vi "ELVIS III v1.0 Block Write DMA.vi"   [LabVIEW 2021]
uses:
  <vilib>/Platform/TimedLoop/XDataNode/timing_clust.ctl
  <vilib>/Platform/TimedLoop/XDataNode/nitl_modes.ctl
  <vilib>/Platform/TimedLoop/XDataNode/wakeup.ctl
  <vilib>/myRIO/Common/Instrument Driver Framework/Utilities/typedefs/FPGA Ref Manager Action Enum.ctl
  <vilib>/myRIO/Common/Instrument Driver Framework/ELVIS III v1.0/DO Block/typedefs/ELVIS III DO Block FPGA Reference.ctl
  <vilib>/myRIO/Common/Instrument Driver Framework/ELVIS III v1.0/AO Block/typedefs/ELVIS III AO Block Channels FPGA Reference.ctl
  <vilib>/Utility/error.llb/Error Cluster From Error Code.vi
  <vilib>/rvi/errors/niLvFpgaAdjustHostInterfaceError.vi
  <vilib>/RVI Host/nirviSupport.llb/nirviErrorClusterFromErrorCode.vi
  <vilib>/platform/TimedLoop/XDataNode/XDataNode.xnode
  <vilib>/myRIO/Common/Instrument Driver Framework/Utilities/typedefs/Generic FPGA Reference.ctl
  <vilib>/rvi/interface/nirviReadWriteControl/nirviReadWriteControl.xnode
  <vilib>/rvi/interface/nirviMethod/nirviMethod.xnode
  <vilib>/Platform/TimedLoop/XDataNode/XDNodeRunTimeDep.lvlib
  <vilib>/rvi/interface/nirviMethod/StockFPGA_InlinedMethodWaitForMultipleIRQ.vi
  <vilib>/FPGAPlugInAG/Dynamic/niLvFpga_WaitOnIrq_Dynamic.vi
  NiFpgaLv.dll
  <vilib>/rvi/interface/Simulation/niFpgaSimulationCallBeginRW.vi
  <vilib>/FPGAPlugInAG/Dynamic/niLvFpga_AcknowledgeIrq_Dynamic.vi
types:
  T1 = typedef "Semaphore RefNum" = refnum<k1>
  T2 = typedef "FPGA Ref Manager Action Enum.ctl" = enum16{"Get", "Set", "Reset"}
  T3 = typedef "Generic FPGA Reference.ctl" = refnum<k20>
  T4 = typedef "XDNodeRunTimeDep.lvlib/timing_clust.ctl" = cluster{"Expected End [f-1]":u64, "Actual End [f-1]":u64, "Finished Late? [f-1]":bool, "Expected End [i-1]":u64, "Actual End [i-1]":u64, "Finished Late? [i-1]":bool, "Expected Start [i]":u64, "Actual Start [i]":u64, "Expected Start [f]":u64, "Actual Start [f]":u64, "Source Name":string, "Structure Name":string, "Period":i64, "Deadline":i64, "Offset":i64, "Start":i64, "Priority":i32, "Timeout":i32, "Mode":T5, "Wakeup Reason":T6, "Error":errorcluster, "Source Type":string, "Secondary Source Type":string, "Global End Time":u64, "Global Start Time":u64, "Frame Duration":u64, "Iteration Duration":u64, "Assigned CPU":i32, "I/O Scan Engine Mode":u32}
  T5 = typedef "XDNodeRunTimeDep.lvlib/nitl_modes.ctl" = enum32{"No Change", "Process missed periods, maintain original phase", "Discard missed periods, maintain original phase", "Process missed periods, ignore original phase", "Discard missed periods, ignore original phase"}
  T6 = typedef "XDNodeRunTimeDep.lvlib/wakeup.ctl" = enum32{"Normal", "Aborted", "Asynchronous wakeup", "Timing source error", "Timed loop error", "Timeout"}
  T7 = typedef "ELVIS III DO Block FPGA Reference.ctl" = refnum<k20>
  T8 = typedef "ELVIS III DO Block Configuration.ctl" = cluster{"Wait Until Done?":bool, "DO FIFO Clock Divisor":u16, "Write Mode":u8, "DO (N Samples) Bank Data ":T9[]}
  T9 = typedef "ELVIS III DO Block Bank Data.ctl" = cluster{"Digital Data Reference":refnum<data-value>, "Channel  Bitmask":fxp<+,20,20>, "Semaphore":T1}
  T10 = typedef "ELVIS III AO Block Channels FPGA Reference.ctl" = refnum<k20>
  T11 = typedef "ELVIS III AO Block Configuration.ctl" = cluster{"AO FIFO Clock Divisor":u32, "Wait Until Done?":bool, "Write Mode":u8, "AO (N Samples) Configuration ":T12[]}
  T12 = typedef "ELVIS III AO Block Bank Data.ctl" = cluster{"Analog data reference":refnum<data-value>, "Semaphore":T1, "ENA_MASK":u8}
  T13 = typedef "Block Write Resource.ctl" = refnum<vi>
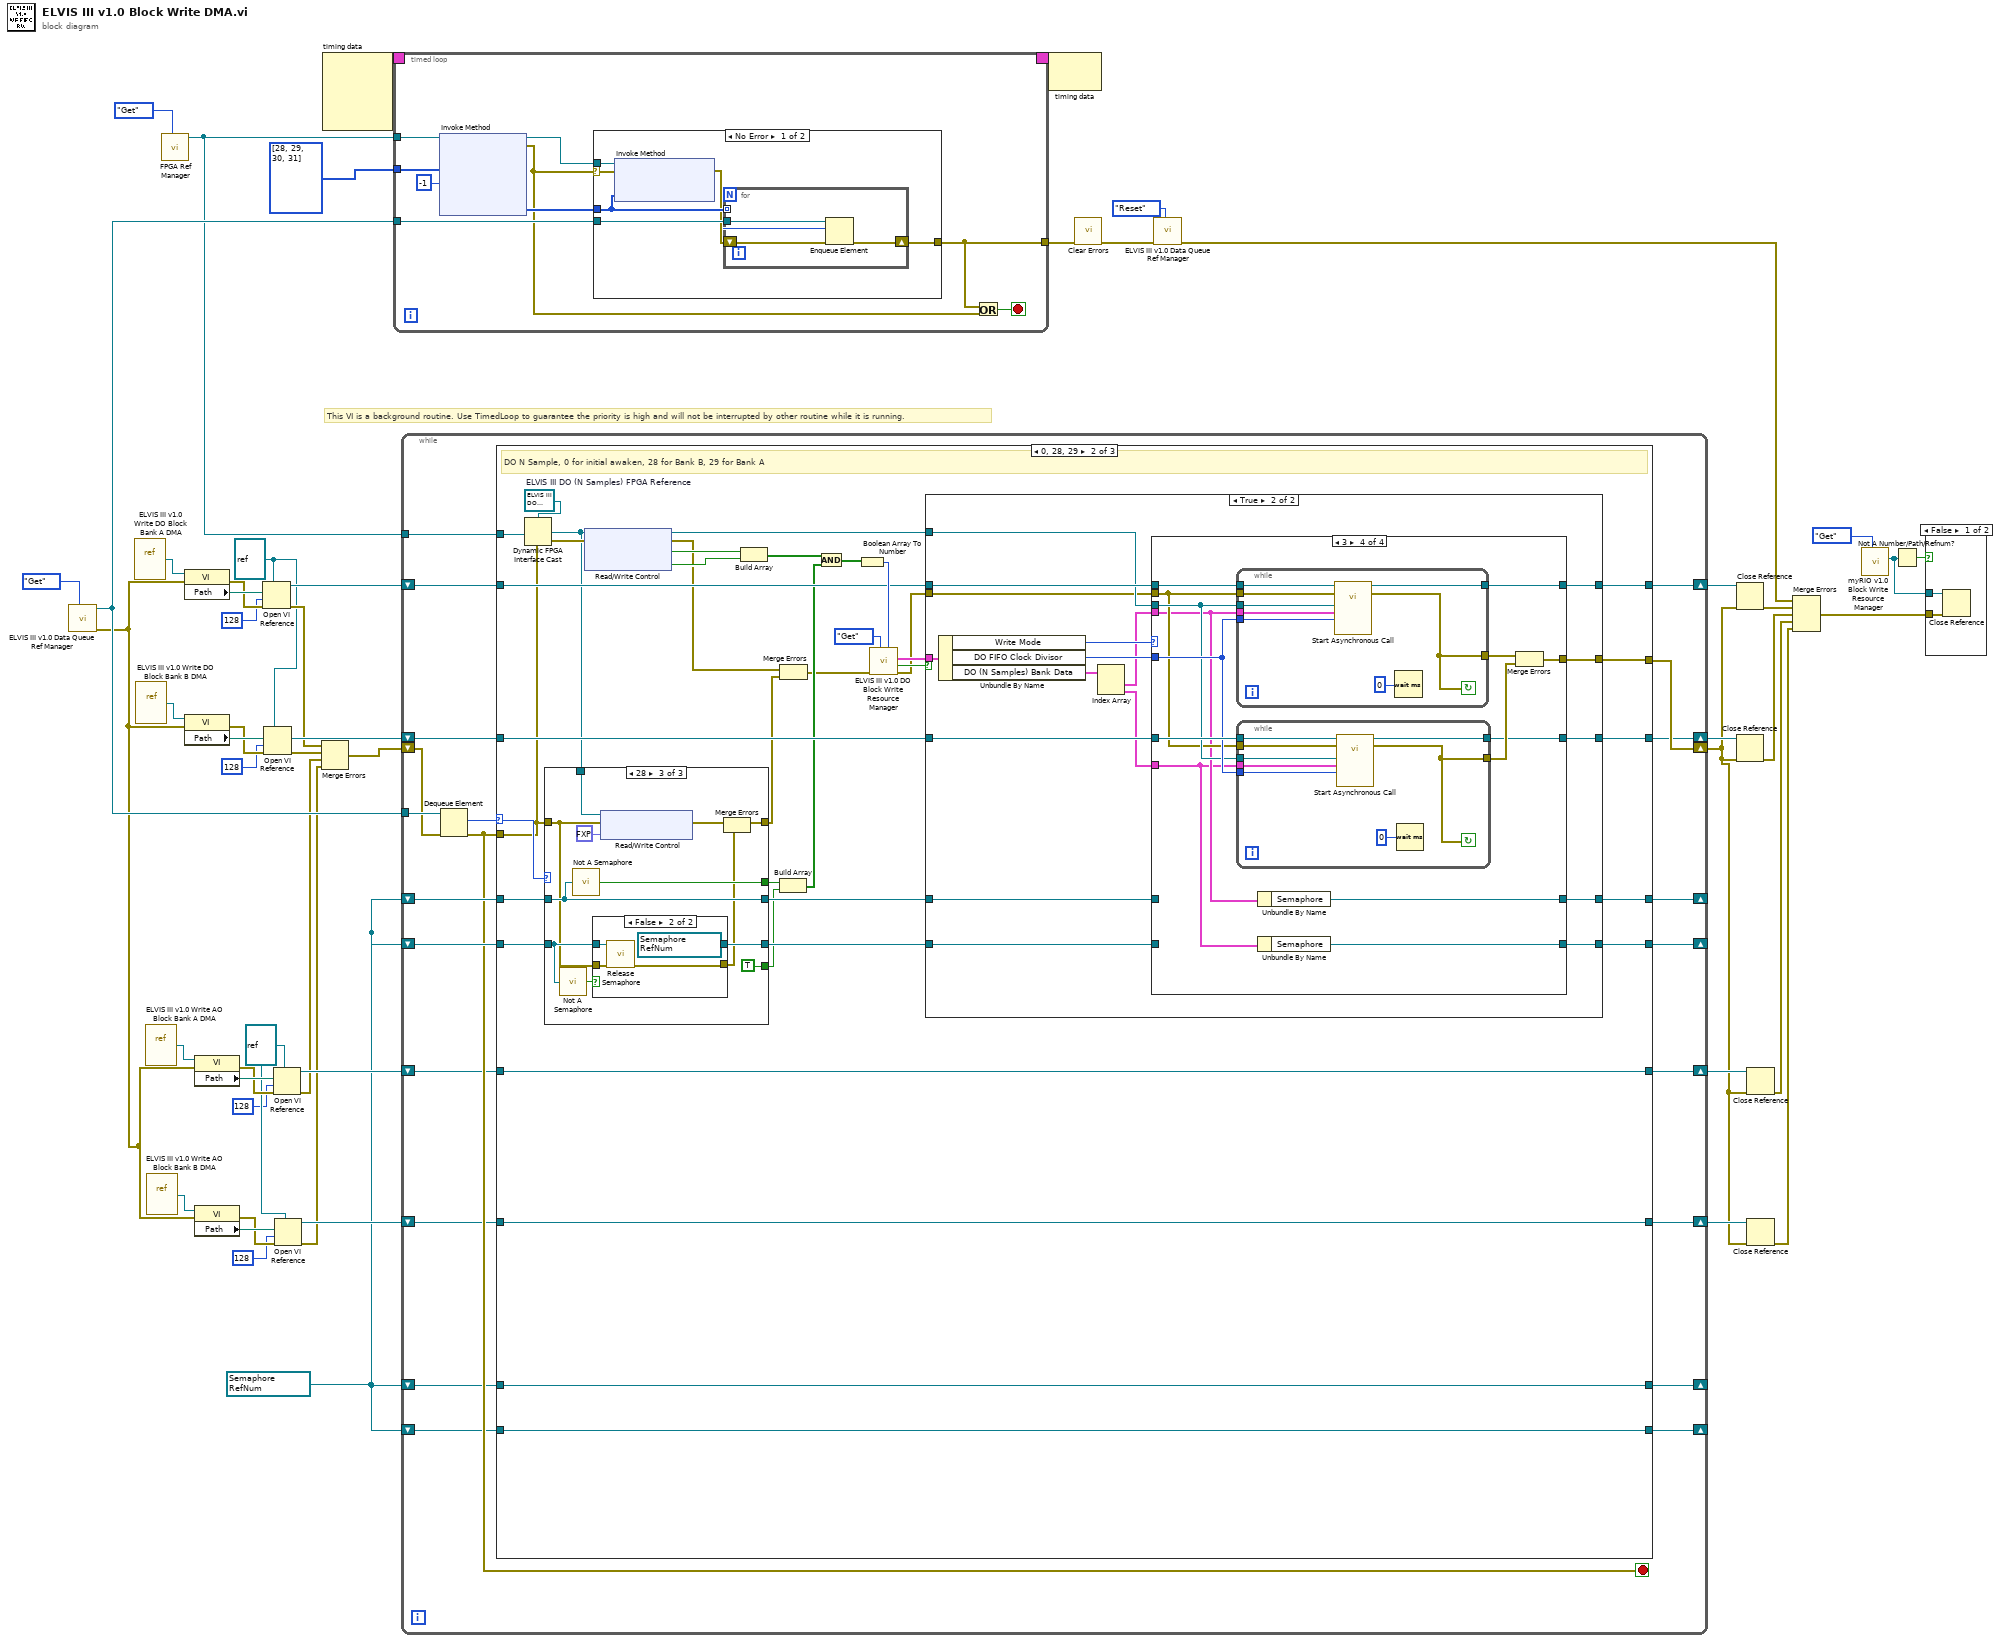
[diagram p0: block diagram]
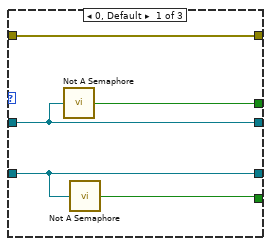
[diagram p4: hidden frame]
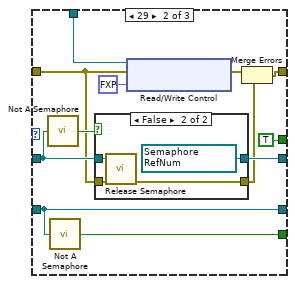
[diagram p5: hidden frame]
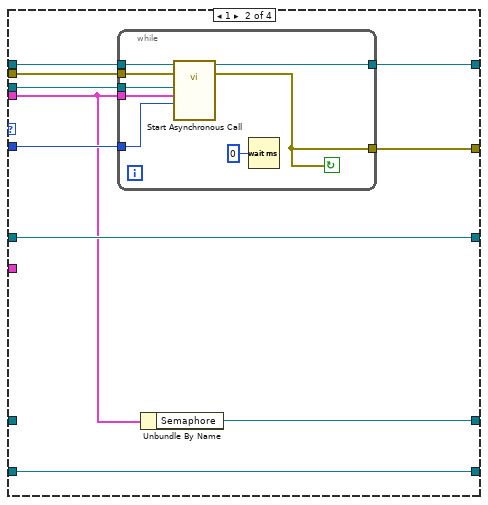
[diagram p10: hidden frame]
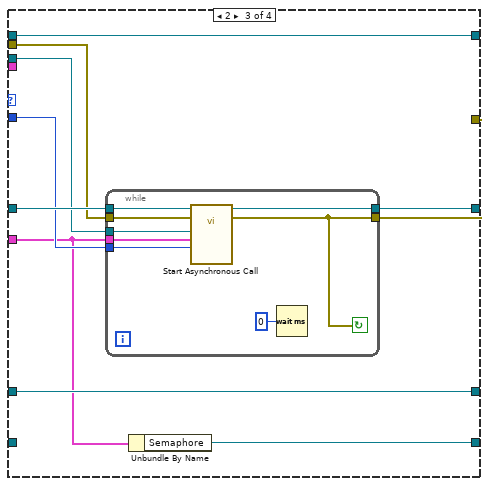
[diagram p11: hidden frame]
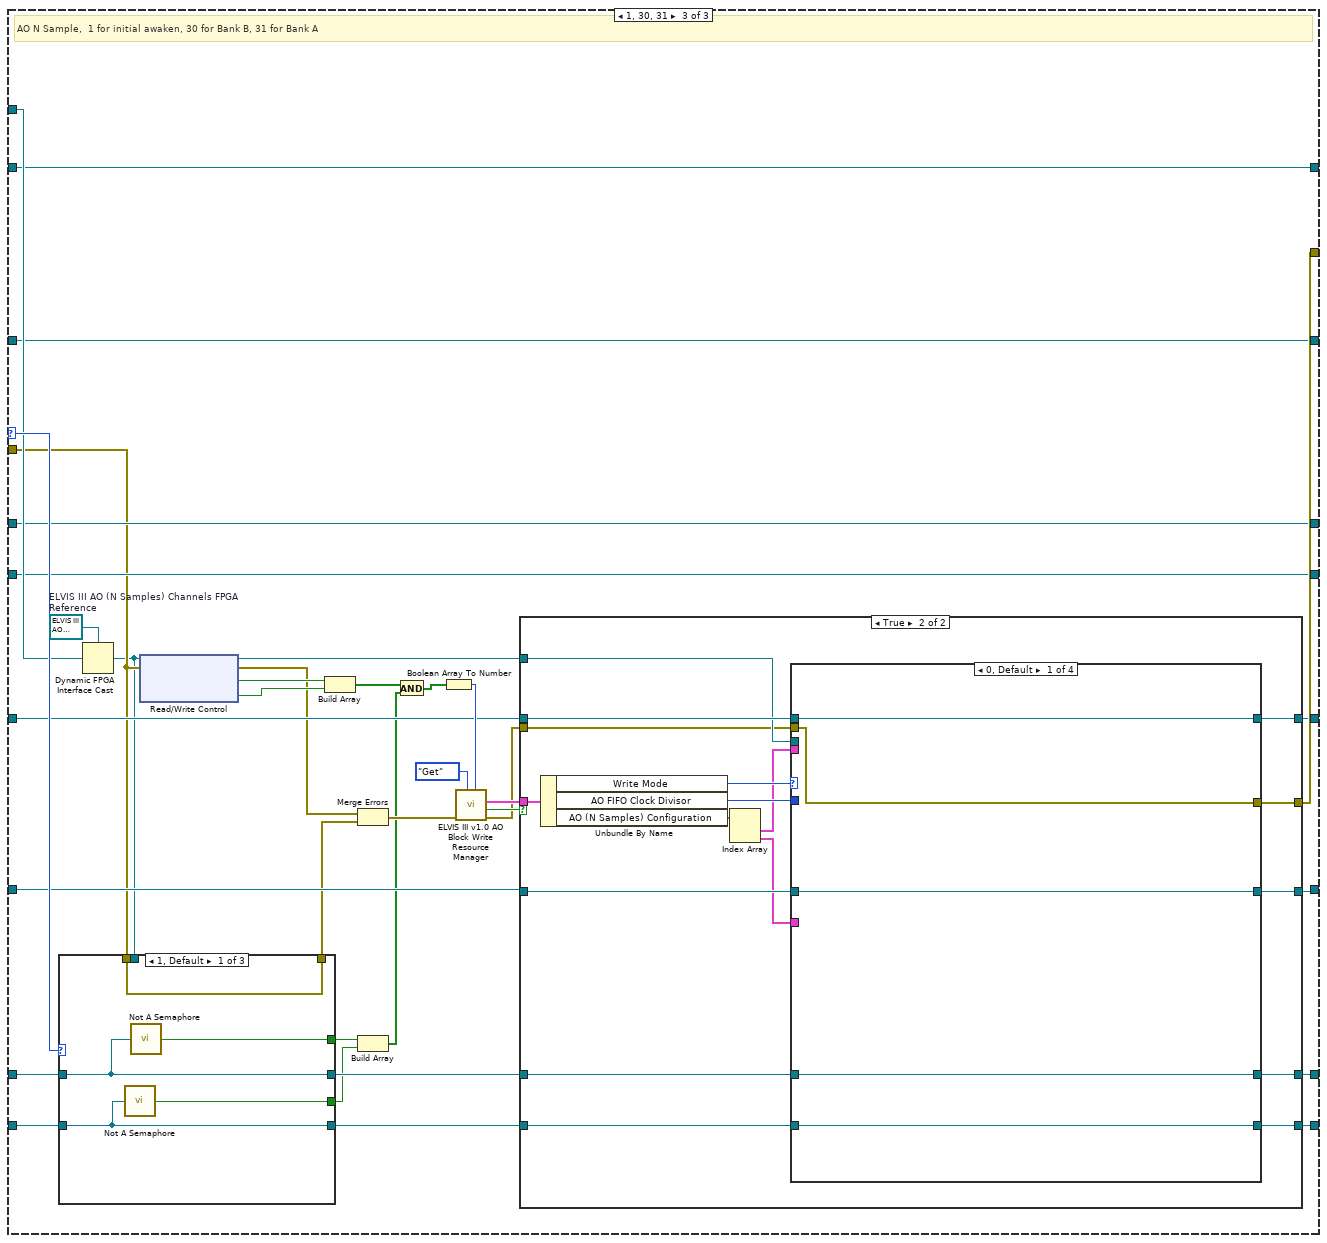
[diagram p12: hidden frame]
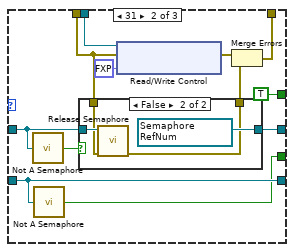
[diagram p13: hidden frame]
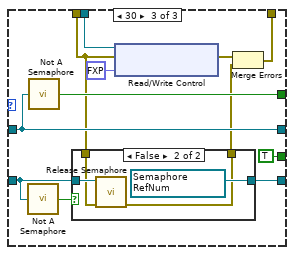
[diagram p15: hidden frame]
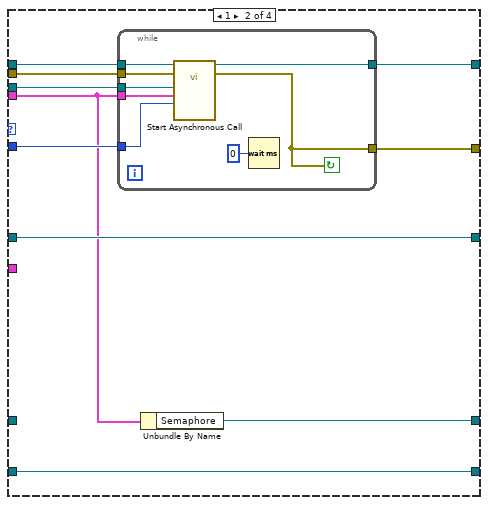
[diagram p18: hidden frame]
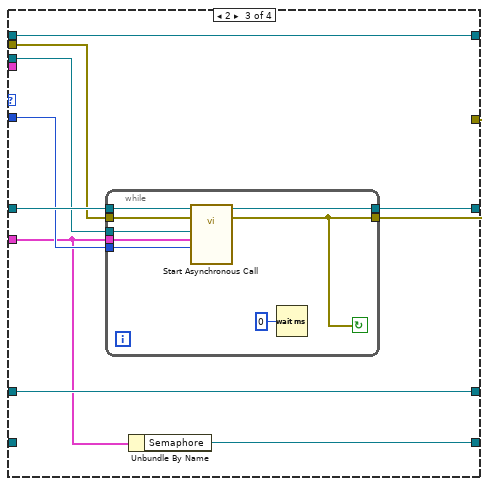
[diagram p19: hidden frame]
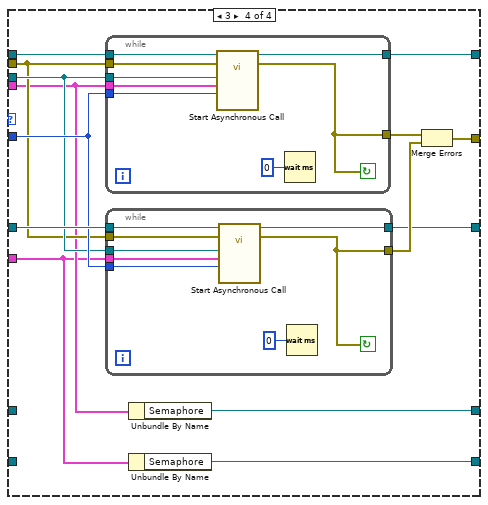
[diagram p20: hidden frame]
diagram:
  w12 = T1 refnum items=["semaphore"] ("Semaphore")
  w24 = refnum<vi> refnum ("type specifier VI Refnum (for type only)")
  w33 = refnum<vi> refnum ("type specifier VI Refnum (for type only)")
  # "This VI is a background routine. Use TimedLoop to guarantee the priority is high and will not be interrupted by other routine while it is running."
  n1 = call <vilib>:"ELVIS III v1.0 Data Queue Ref Manager.vi"("Action"=enum16{"Get", "Reset"}."Get") -> ("error out"=w21:errorcluster, "Queue out"=w48:refnum<queue>)  [unwired: 8 in]
  n2 = vi-ref <vilib>:"ELVIS III v1.0 Write DO Block Bank A DMA.vi"() -> (w47:refnum<vi>)
  n3 = vi-ref <vilib>:"ELVIS III v1.0 Write DO Block Bank B DMA.vi"() -> (w45:refnum<vi>)
  n4 = vi-ref <vilib>:"ELVIS III v1.0 Write AO Block Bank A DMA.vi"() -> (w30:refnum<vi>)
  n5 = vi-ref <vilib>:"ELVIS III v1.0 Write AO Block Bank B DMA.vi"() -> (w28:refnum<vi>)
  n6 = call <vilib>:"FPGA Ref Manager.vi"("Action"=FPGA_Ref_Manager_Action_Enum."Get") -> ("Generic FPGA Reference out"=w36:T3)  [unwired: 8 in, 1 out]
  n7 = property class="VI"(reference=w47, error in=w21) -> (error out=w42:errorcluster, "Path"=w46:path)  [unwired: 1 out]
  n8 = property class="VI"(reference=w45, error in=w21) -> (error out=w40:errorcluster, "Path"=w44:path)  [unwired: 1 out]
  n9 = property class="VI"(reference=w30, error in=w21) -> (error out=w26:errorcluster, "Path"=w29:path)  [unwired: 1 out]
  n10 = property class="VI"(reference=w28, error in=w21) -> (error out=w25:errorcluster, "Path"=w27:path)  [unwired: 1 out]
  n11 = Open VI Reference(type specifier VI Refnum (for type only)=w33, vi path=w46, options=128, error in (no error)=w42) -> (vi reference=w43:refnum<vi>, error out=w39:errorcluster)  [unwired: 2 in]
  n12 = Open VI Reference(type specifier VI Refnum (for type only)=w33, vi path=w44, options=128, error in (no error)=w40) -> (vi reference=w41:refnum<vi>, error out=w38:errorcluster)  [unwired: 2 in]
  n13 = Open VI Reference(type specifier VI Refnum (for type only)=w24, vi path=w29, options=128, error in (no error)=w26) -> (vi reference=w20:refnum<vi>, error out=w15:errorcluster)  [unwired: 2 in]
  n14 = Open VI Reference(type specifier VI Refnum (for type only)=w24, vi path=w27, options=128, error in (no error)=w25) -> (vi reference=w19:refnum<vi>, error out=w14:errorcluster)  [unwired: 2 in]
  n15 = Merge Errors(w39, w38, w15, w14) -> (w37:errorcluster)
  n16 = node-c288() -> (w53:T4)  [unwired: 4 in]
  n17 = timed-loop {
    timing: w53 -> [_]
    timing-out: [_] -> w52
    tunnel: i32[] [28, 29, 30, 31] -> [w62]
    tunnel: w48 -> [w59]
    tunnel: w36 -> [w57]
    tunnel: [w54] -> w13
    stop <- w55 stop-if-true
    n18 = xnode "Invoke Method"("FPGA VI Reference In"=w57, "IRQ Number(s)"=w62, "Timeout (ms)"=-1) -> ("FPGA VI Reference Out"=w56:T3, "error out"=w58:errorcluster, "IRQ(s) Asserted"=w60:i32[])  [unwired: 1 in, 1 out]
    n19 = case shown="No Error" w58 {
      selector: w58 -> [w64 w73]
      tunnel: w60 -> [w66 _]
      tunnel: w59 -> [w68 _]
      tunnel: [w67 w73] -> w54
      tunnel: w56 -> [w65 _]
      frame No Error {
        n20 = xnode "Invoke Method"("FPGA VI Reference In"=w65, "error in"=w64, "IRQ Number(s)"=w66) -> ("error out"=w63:errorcluster)  [unwired: 1 out]
        n21 = for {
          tunnel: w66 -> [w69] mode=indexing
          tunnel: w68 -> [w72]
          shift-right: [w70] -> w67
          shift-left: w63 -> [w71]
          n22 = Enqueue Element(queue=w72, element=w69, error in (no error)=w71) -> (error out=w70:errorcluster)  [unwired: 1 in, 2 out]
        }
      }
      frame Error {
      }
    }
    n23 = Or(x=w54, y=w58) -> (x .or. y?=w55:bool)
  }
  n24 = while {
    tunnel: w48 -> [w97]
    shift-right: [w90] -> w35
    shift-left: w43 -> [w93]
    shift-right: [w91] -> w34
    shift-left: w41 -> [w94]
    shift-right: [w92] -> w16
    shift-left: w37 -> [w95]
    shift-right: [w87] -> _
    shift-left: w12 -> [w89]
    shift-right: [w86] -> _
    shift-left: w12 -> [w88]
    tunnel: w36 -> [w84]
    shift-right: [w79] -> _
    shift-left: w12 -> [w83]
    shift-right: [w78] -> _
    shift-left: w12 -> [w82]
    shift-right: [w77] -> w18
    shift-left: w20 -> [w81]
    shift-right: [w76] -> w17
    shift-left: w19 -> [w80]
    stop <- w85 stop-if-true
    n25 = Dequeue Element(queue=w97, error in (no error)=w95) -> (element=w96:i32, error out=w85:errorcluster)  [unwired: 1 in, 2 out]
    n26 = case shown="0, 28, 29" w96 {
      selector: w96 -> [_ w132 w306]
      tunnel: w85 -> [w104 w111 w286]
      tunnel: w94 -> [w105 w134 w289]
      tunnel: w93 -> [w106 w135 w290]
      tunnel: [w104 w140 w312] -> w92
      tunnel: [w105 w141 w289] -> w91
      tunnel: [w106 w142 w290] -> w90
      tunnel: w89 -> [w103 w131 w294]
      tunnel: w88 -> [w102 w130 w293]
      tunnel: [w103 w129 w294] -> w87
      tunnel: [w102 w128 w293] -> w86
      tunnel: w84 -> [_ w124 w302]
      tunnel: w83 -> [w101 w118 w298]
      tunnel: w82 -> [w100 w117 w297]
      tunnel: w81 -> [w99 w120 w296]
      tunnel: w80 -> [w98 w119 w295]
      tunnel: [w101 w118 w292] -> w79
      tunnel: [w100 w117 w291] -> w78
      tunnel: [w99 w120 w288] -> w77
      tunnel: [w98 w119 w287] -> w76
      frame Default {
      }
      frame 0, 28, 29 {
        w125 = T7 refnum  # ELVIS III DO (N Samples) FPGA Reference
        # "DO N Sample, 0 for initial awaken, 28 for Bank B, 29 for Bank A"
        n27 = Dynamic FPGA Interface Cast(Session In=w125, Type=w124) -> (Session Out=w110:T7)
        n28 = case shown="28" w132 {
          tunnel: w131 -> [w145 w155 w173]
          tunnel: w130 -> [w144 w153 w171]
          tunnel: [w144 w153 w177] -> w127
          tunnel: [w145 w159 w173] -> w126
          tunnel: [w146 TRUE w172] -> w116
          tunnel: [w143 w152 TRUE] -> w115
          tunnel: w111 -> [w147 w151 w169]
          tunnel: w110 -> [_ w156 w174]
          tunnel: [w147 w149 w166] -> w109
          frame 0, Default {
            n29 = call <vilib>:"Not A Semaphore.vi"("semaphore"=w145) -> ("not a semaphore"=w146:bool)
            n30 = call <vilib>:"Not A Semaphore.vi"("semaphore"=w144) -> ("not a semaphore"=w143:bool)
          }
          frame 29 {
            n31 = call <vilib>:"Not A Semaphore.vi"("semaphore"=w155) -> ("not a semaphore"=w154:bool)
            n32 = call <vilib>:"Not A Semaphore.vi"("semaphore"=w153) -> ("not a semaphore"=w152:bool)
            n33 = case shown="False" w154 {
              tunnel: w155 -> [w161 w165]
              tunnel: [w161 w164] -> w159
              tunnel: w151 -> [w160 w163]
              tunnel: [w160 w162] -> w148
              frame True {
              }
              frame False {
                w164 = T1 refnum items=["semaphore"] ("Semaphore")
                n34 = call <vilib>:"Release Semaphore.vi"("error in (no error)"=w163, "semaphore"=w165) -> ("error out"=w162:errorcluster)  [unwired: 4 in, 1 out]
              }
            }
            n35 = xnode "Read/Write Control"("FPGA VI Reference In"=w156, "error in"=w151, "DO.A.DMA_ENA"=fxp<+,20,20> 0.0) -> ("error out"=w150:errorcluster)  [unwired: 1 out]
            n36 = Merge Errors(w150, w148) -> (w149:errorcluster)
          }
          frame 28 {
            n37 = call <vilib>:"Not A Semaphore.vi"("semaphore"=w171) -> ("not a semaphore"=w170:bool)
            n38 = call <vilib>:"Not A Semaphore.vi"("semaphore"=w173) -> ("not a semaphore"=w172:bool)
            n39 = case shown="False" w170 {
              tunnel: w171 -> [w179 w183]
              tunnel: [w179 w182] -> w177
              tunnel: w169 -> [w178 w181]
              tunnel: [w178 w180] -> w167
              frame True {
              }
              frame False {
                w182 = T1 refnum items=["semaphore"] ("Semaphore")
                n40 = call <vilib>:"Release Semaphore.vi"("error in (no error)"=w181, "semaphore"=w183) -> ("error out"=w180:errorcluster)  [unwired: 4 in, 1 out]
              }
            }
            n41 = xnode "Read/Write Control"("FPGA VI Reference In"=w174, "error in"=w169, "DO.B.DMA_ENA"=fxp<+,20,20> 0.0 ("DO.A.DMA_ENA")) -> ("error out"=w168:errorcluster)  [unwired: 1 out]
            n42 = Merge Errors(w168, w167) -> (w166:errorcluster)
          }
        }
        n43 = xnode "Read/Write Control"("FPGA VI Reference In"=w110, "error in"=w111) -> ("FPGA VI Reference Out"=w122:T7, "error out"=w108:errorcluster, "DO.A.DMA_IDL"=w139:bool, "DO.B.DMA_IDL"=w138:bool)
        n44 = Build Array(w139, w138) -> (w114:bool[])
        n45 = Build Array(w116, w115) -> (w113:bool[])
        n46 = Merge Errors(w108, w109) -> (w107:errorcluster)
        n47 = And(x=w114, y=w113) -> (x .and. y?=w112:bool[])
        n48 = Boolean Array To Number(Boolean array=w112) -> (number=w137:u8)
        n49 = call <vilib>:"ELVIS III v1.0 DO Block Write Resource Manager.vi"("DMA Resource"=w137, "Action"=enum16{"Set", "Get"}."Get", "error in (no error)"=w107) -> ("error out"=w121:errorcluster, "Action Succeeds"=w136:bool, "DO Resource Out"=w133:T8)  [unwired: 6 in]
        n50 = case shown="True" w136 {
          tunnel: w135 -> [w188 w205]
          tunnel: [w188 w204] -> w142
          tunnel: [w187 w203] -> w141
          tunnel: w134 -> [w187 w202]
          tunnel: [w184 w201] -> w140
          tunnel: w133 -> [_ w195]
          tunnel: [w186 w200] -> w129
          tunnel: [w185 w199] -> w128
          tunnel: w127 -> [w185 w198]
          tunnel: w126 -> [w186 w197]
          tunnel: w122 -> [_ w192]
          tunnel: w121 -> [w184 w189]
          frame False {
          }
          frame True {
            n51 = Unbundle By Name(w195) -> ("Write Mode"=w194:u8, "DO FIFO Clock Divisor"=w193:u16, "DO (N Samples) Bank Data"=w196:T9[])
            n52 = Index Array(array=w196) -> (element #1=w190:T9, element #2=w191:T9)  [unwired: 2 in]
            n53 = case shown="3" w194 {
              tunnel: w205 -> [w210 w220 w234 w260]
              tunnel: [w210 w218 w234 w255] -> w204
              tunnel: [w209 w217 w236 w254] -> w203
              tunnel: w202 -> [w209 w217 w238 w259]
              tunnel: w189 -> [w208 w213 w237 w251]
              tunnel: [w208 w216 w235 w258] -> w201
              tunnel: [w207 w211 w233 w249] -> w200
              tunnel: [w206 w219 w229 w247] -> w199
              tunnel: w198 -> [w206 w219 _ _]
              tunnel: w197 -> [w207 _ w233 _]
              tunnel: w193 -> [_ w214 w231 w253]
              tunnel: w192 -> [_ w215 w232 w252]
              tunnel: w191 -> [_ _ w230 w248]
              tunnel: w190 -> [_ w212 _ w250]
              frame 0, Default {
              }
              frame 1 {
                n54 = while {
                  tunnel: w220 -> [w227]
                  tunnel: [w223] -> w218
                  tunnel: [w222] -> w216
                  tunnel: w215 -> [w226]
                  tunnel: w212 -> [w225]
                  tunnel: w214 -> [w224]
                  tunnel: w213 -> [w221]
                  stop <- w222 continue-if-true
                  n55 = call-by-ref "Start Asynchronous Call"(reference=w227, error in=w221, "DO FIFO Clock Divisor"=w224, "Bank Data"=w225, "FPGA Reference out"=w226) -> (reference out=w223:refnum<vi>, error out=w222:errorcluster)  [unwired: 8 in, 1 out]
                  n56 = Wait (ms)(milliseconds to wait=u32 0) -> ()  [unwired: 1 out]
                }
                n57 = Unbundle By Name(w212) -> ("Semaphore"=w211:T1)
              }
              frame 2 {
                n58 = while {
                  tunnel: w238 -> [w245]
                  tunnel: w237 -> [w244]
                  tunnel: [w243] -> w236
                  tunnel: [w242] -> w235
                  tunnel: w230 -> [w241]
                  tunnel: w232 -> [w240]
                  tunnel: w231 -> [w239]
                  stop <- w242 continue-if-true
                  n59 = call-by-ref "Start Asynchronous Call"(reference=w245, error in=w244, "DO FIFO Clock Divisor"=w239, "Bank Data"=w241, "FPGA Reference out"=w240) -> (reference out=w243:refnum<vi>, error out=w242:errorcluster)  [unwired: 8 in, 1 out]
                  n60 = Wait (ms)(milliseconds to wait=u32 0) -> ()  [unwired: 1 out]
                }
                n61 = Unbundle By Name(w230) -> ("Semaphore"=w229:T1)
              }
              frame 3 {
                n62 = while {
                  tunnel: w260 -> [w275]
                  tunnel: w251 -> [w273]
                  tunnel: [w274] -> w255
                  tunnel: [w272] -> w257
                  tunnel: w253 -> [w271]
                  tunnel: w252 -> [w270]
                  tunnel: w250 -> [w269]
                  stop <- w272 continue-if-true
                  n63 = call-by-ref "Start Asynchronous Call"(reference=w275, error in=w273, "DO FIFO Clock Divisor"=w271, "Bank Data"=w269, "FPGA Reference out"=w270) -> (reference out=w274:refnum<vi>, error out=w272:errorcluster)  [unwired: 8 in, 1 out]
                  n64 = Wait (ms)(milliseconds to wait=u32 0) -> ()  [unwired: 1 out]
                }
                n65 = while {
                  tunnel: w259 -> [w267]
                  tunnel: w251 -> [w266]
                  tunnel: [w264] -> w254
                  tunnel: [w265] -> w256
                  tunnel: w253 -> [w263]
                  tunnel: w252 -> [w262]
                  tunnel: w248 -> [w261]
                  stop <- w265 continue-if-true
                  n66 = call-by-ref "Start Asynchronous Call"(reference=w267, error in=w266, "DO FIFO Clock Divisor"=w263, "Bank Data"=w261, "FPGA Reference out"=w262) -> (reference out=w264:refnum<vi>, error out=w265:errorcluster)  [unwired: 8 in, 1 out]
                  n67 = Wait (ms)(milliseconds to wait=u32 0) -> ()  [unwired: 1 out]
                }
                n68 = Unbundle By Name(w250) -> ("Semaphore"=w249:T1)
                n69 = Unbundle By Name(w248) -> ("Semaphore"=w247:T1)
                n70 = Merge Errors(w257, w256) -> (w258:errorcluster)
              }
            }
          }
        }
      }
      frame 1, 30, 31 {
        w303 = T10 refnum  # ELVIS III AO (N Samples) Channels FPGA Reference
        # "AO N Sample,  1 for initial awaken, 30 for Bank B, 31 for Bank A"
        n71 = Dynamic FPGA Interface Cast(Session In=w303, Type=w302) -> (Session Out=w285:T10)
        n72 = case shown="1, Default" w306 {
          tunnel: w298 -> [w315 w325 w342]
          tunnel: w297 -> [w313 w323 w341]
          tunnel: [w313 w323 w344] -> w305
          tunnel: [w315 w329 w342] -> w304
          tunnel: w286 -> [w317 w321 w339]
          tunnel: w285 -> [_ w327 w346]
          tunnel: [w317 w318 w337] -> w283
          tunnel: [w316 TRUE w343] -> w281
          tunnel: [w314 w322 TRUE] -> w280
          frame 1, Default {
            n73 = call <vilib>:"Not A Semaphore.vi"("semaphore"=w313) -> ("not a semaphore"=w314:bool)
            n74 = call <vilib>:"Not A Semaphore.vi"("semaphore"=w315) -> ("not a semaphore"=w316:bool)
          }
          frame 31 {
            n75 = call <vilib>:"Not A Semaphore.vi"("semaphore"=w325) -> ("not a semaphore"=w324:bool)
            n76 = call <vilib>:"Not A Semaphore.vi"("semaphore"=w323) -> ("not a semaphore"=w322:bool)
            n77 = case shown="False" w324 {
              tunnel: w325 -> [w331 w335]
              tunnel: [w331 w334] -> w329
              tunnel: w321 -> [w330 w333]
              tunnel: [w330 w332] -> w319
              frame True {
              }
              frame False {
                w334 = T1 refnum items=["semaphore"] ("Semaphore")
                n78 = call <vilib>:"Release Semaphore.vi"("error in (no error)"=w333, "semaphore"=w335) -> ("error out"=w332:errorcluster)  [unwired: 4 in, 1 out]
              }
            }
            n79 = xnode "Read/Write Control"("FPGA VI Reference In"=w327, "error in"=w321, "AO.A.DMA_ENA"=fxp<+,2,2> 0.0 ("AO.B.DMA_ENA")) -> ("error out"=w320:errorcluster)  [unwired: 1 out]
            n80 = Merge Errors(w320, w319) -> (w318:errorcluster)
          }
          frame 30 {
            n81 = call <vilib>:"Not A Semaphore.vi"("semaphore"=w341) -> ("not a semaphore"=w340:bool)
            n82 = call <vilib>:"Not A Semaphore.vi"("semaphore"=w342) -> ("not a semaphore"=w343:bool)
            n83 = case shown="False" w340 {
              tunnel: w341 -> [w349 w353]
              tunnel: [w349 w352] -> w344
              tunnel: w339 -> [w348 w351]
              tunnel: [w348 w350] -> w336
              frame True {
              }
              frame False {
                w352 = T1 refnum items=["semaphore"] ("Semaphore")
                n84 = call <vilib>:"Release Semaphore.vi"("error in (no error)"=w351, "semaphore"=w353) -> ("error out"=w350:errorcluster)  [unwired: 4 in, 1 out]
              }
            }
            n85 = xnode "Read/Write Control"("FPGA VI Reference In"=w346, "error in"=w339, "AO.B.DMA_ENA"=fxp<+,2,2> 0.0) -> ("error out"=w338:errorcluster)  [unwired: 1 out]
            n86 = Merge Errors(w338, w336) -> (w337:errorcluster)
          }
        }
        n87 = xnode "Read/Write Control"("FPGA VI Reference In"=w285, "error in"=w286) -> ("FPGA VI Reference Out"=w300:T10, "error out"=w284:errorcluster, "AO.A.DMA_IDL"=w311:bool, "AO.B.DMA_IDL"=w310:bool)
        n88 = Build Array(w311, w310) -> (w279:bool[])
        n89 = Merge Errors(w284, w283) -> (w282:errorcluster)
        n90 = Build Array(w281, w280) -> (w278:bool[])
        n91 = And(x=w279, y=w278) -> (x .and. y?=w277:bool[])
        n92 = Boolean Array To Number(Boolean array=w277) -> (number=w309:u8)
        n93 = call <vilib>:"ELVIS III v1.0 AO Block Write Resource Manager.vi"("DMA Resource"=w309, "Action"=enum16{"Set", "Get"}."Get", "error in (no error)"=w282) -> ("error out"=w299:errorcluster, "Action Succeeds"=w308:bool, "AO Resource Out"=w307:T11)  [unwired: 6 in]
        n94 = case shown="True" w308 {
          tunnel: w296 -> [w358 w375]
          tunnel: [w358 w374] -> w288
          tunnel: [w357 w373] -> w287
          tunnel: w295 -> [w357 w372]
          tunnel: [w354 w371] -> w312
          tunnel: w307 -> [_ w365]
          tunnel: [w356 w370] -> w292
          tunnel: [w355 w369] -> w291
          tunnel: w305 -> [w355 w368]
          tunnel: w304 -> [w356 w367]
          tunnel: w300 -> [_ w362]
          tunnel: w299 -> [w354 w359]
          frame False {
          }
          frame True {
            n95 = Unbundle By Name(w365) -> ("Write Mode"=w364:u8, "AO FIFO Clock Divisor"=w363:u32, "AO (N Samples) Configuration"=w366:T12[])
            n96 = Index Array(array=w366) -> (element #1=w360:T12, element #2=w361:T12)  [unwired: 2 in]
            n97 = case shown="0, Default" w364 {
              tunnel: w375 -> [w380 w390 w404 w430]
              tunnel: [w380 w388 w404 w425] -> w374
              tunnel: [w379 w387 w406 w424] -> w373
              tunnel: w372 -> [w379 w387 w408 w429]
              tunnel: w359 -> [w378 w383 w407 w421]
              tunnel: [w378 w386 w405 w428] -> w371
              tunnel: [w377 w381 w403 w419] -> w370
              tunnel: [w376 w389 w399 w417] -> w369
              tunnel: w368 -> [w376 w389 _ _]
              tunnel: w367 -> [w377 _ w403 _]
              tunnel: w363 -> [_ w384 w401 w423]
              tunnel: w362 -> [_ w385 w402 w422]
              tunnel: w361 -> [_ _ w400 w418]
              tunnel: w360 -> [_ w382 _ w420]
              frame 0, Default {
              }
              frame 1 {
                n98 = while {
                  tunnel: w390 -> [w397]
                  tunnel: [w394] -> w388
                  tunnel: [w393] -> w386
                  tunnel: w385 -> [w396]
                  tunnel: w382 -> [w391]
                  tunnel: w384 -> [w395]
                  tunnel: w383 -> [w392]
                  stop <- w393 continue-if-true
                  n99 = call-by-ref "Start Asynchronous Call"(reference=w397, error in=w392, "AO FIFO Clock Divisor"=w395, "Bank Data"=w391, "FPGA Reference out"=w396) -> (reference out=w394:refnum<vi>, error out=w393:errorcluster)  [unwired: 8 in, 1 out]
                  n100 = Wait (ms)(milliseconds to wait=u32 0) -> ()  [unwired: 1 out]
                }
                n101 = Unbundle By Name(w382) -> ("Semaphore"=w381:T1)
              }
              frame 2 {
                n102 = while {
                  tunnel: w408 -> [w415]
                  tunnel: w407 -> [w414]
                  tunnel: [w413] -> w406
                  tunnel: [w412] -> w405
                  tunnel: w400 -> [w409]
                  tunnel: w402 -> [w411]
                  tunnel: w401 -> [w410]
                  stop <- w412 continue-if-true
                  n103 = call-by-ref "Start Asynchronous Call"(reference=w415, error in=w414, "AO FIFO Clock Divisor"=w410, "Bank Data"=w409, "FPGA Reference out"=w411) -> (reference out=w413:refnum<vi>, error out=w412:errorcluster)  [unwired: 8 in, 1 out]
                  n104 = Wait (ms)(milliseconds to wait=u32 0) -> ()  [unwired: 1 out]
                }
                n105 = Unbundle By Name(w400) -> ("Semaphore"=w399:T1)
              }
              frame 3 {
                n106 = while {
                  tunnel: w430 -> [w440]
                  tunnel: w421 -> [w444]
                  tunnel: [w445] -> w425
                  tunnel: [w443] -> w427
                  tunnel: w423 -> [w442]
                  tunnel: w422 -> [w441]
                  tunnel: w420 -> [w439]
                  stop <- w443 continue-if-true
                  n107 = call-by-ref "Start Asynchronous Call"(reference=w440, error in=w444, "AO FIFO Clock Divisor"=w442, "Bank Data"=w439, "FPGA Reference out"=w441) -> (reference out=w445:refnum<vi>, error out=w443:errorcluster)  [unwired: 8 in, 1 out]
                  n108 = Wait (ms)(milliseconds to wait=u32 0) -> ()  [unwired: 1 out]
                }
                n109 = while {
                  tunnel: w429 -> [w437]
                  tunnel: w421 -> [w436]
                  tunnel: [w434] -> w424
                  tunnel: [w435] -> w426
                  tunnel: w423 -> [w433]
                  tunnel: w422 -> [w432]
                  tunnel: w418 -> [w431]
                  stop <- w435 continue-if-true
                  n110 = call-by-ref "Start Asynchronous Call"(reference=w437, error in=w436, "AO FIFO Clock Divisor"=w433, "Bank Data"=w431, "FPGA Reference out"=w432) -> (reference out=w434:refnum<vi>, error out=w435:errorcluster)  [unwired: 8 in, 1 out]
                  n111 = Wait (ms)(milliseconds to wait=u32 0) -> ()  [unwired: 1 out]
                }
                n112 = Unbundle By Name(w420) -> ("Semaphore"=w419:T1)
                n113 = Unbundle By Name(w418) -> ("Semaphore"=w417:T1)
                n114 = Merge Errors(w427, w426) -> (w428:errorcluster)
              }
            }
          }
        }
      }
    }
  }
  n115 = node-c288(w52) -> ()  [unwired: 1 out]
  n116 = call <vilib>:"Clear Errors.vi"("error in (no error)"=w13) -> ("error out"=w2:errorcluster)  [unwired: 5 in, 1 out]
  n117 = call <vilib>:"ELVIS III v1.0 Data Queue Ref Manager.vi"("Action"=enum16{"Get", "Reset"}."Reset", "error in (no error)"=w2) -> ("error out"=w1:errorcluster)  [unwired: 7 in, 1 out]
  n118 = Close Reference(reference=w35, error in (no error)=w16) -> (error out=w8:errorcluster)
  n119 = Close Reference(reference=w34, error in (no error)=w16) -> (error out=w7:errorcluster)
  n120 = Close Reference(reference=w18, error in (no error)=w16) -> (error out=w6:errorcluster)
  n121 = Close Reference(reference=w17, error in (no error)=w16) -> (error out=w5:errorcluster)
  n122 = Merge Errors(w1, w8, w7, w6, w5) -> (w4:errorcluster)
  n123 = call <vilib>:"myRIO v1.0 Block Write Resource Manager.vi"("Action"=enum16{"Get", "Set", "Reset"}."Get") -> ("Resource Data Out"=w9:T13)  [unwired: 10 in]
  n124 = Not A Number/Path/Refnum?(number/path/refnum=w9) -> (NaN/Path/Refnum?=w10:bool)
  n125 = case shown="False" w10 {
    tunnel: w4 -> [w447 _]
    tunnel: w9 -> [w448 _]
    frame False {
      n126 = Close Reference(reference=w448, error in (no error)=w447) -> ()  [unwired: 1 out]
    }
    frame True {
    }
  }
